vi "AuthSrpVerificationRequest_Create.vi"(7 "Header":T3, 8 "error in (no error)":errorcluster, 9 "AuthSrpVerificationRequest":T1, 10 "IRoutingSource":T2, 11 "ReplyTo":string) -> (0 "error out":errorcluster, 3 "Message":T5)   [LabVIEW 2017]
uses:
  <vilib>/addons/InsightCM/MessageBus/Base/controls/Message.ctl
  <vilib>/addons/InsightCM/MessageBus/Base/controls/MessageHeader.ctl
  <vilib>/addons/InsightCM/MessageBus/Base/controls/KeyValuePair.ctl
  <vilib>/addons/InsightCM/MessageBus/Base/controls/IRoutingSource.ctl
  <vilib>/addons/InsightCM/MessageBus/MessageLibrary/Authentication/controls/AuthSrpVerificationRequestBody.ctl
  <vilib>/addons/InsightCM/MessageBus/Base/controls/MessageClassType.ctl
  <vilib>/addons/InsightCM/Utilities/PropertyHelpers/PropertyHelpers.lvlib
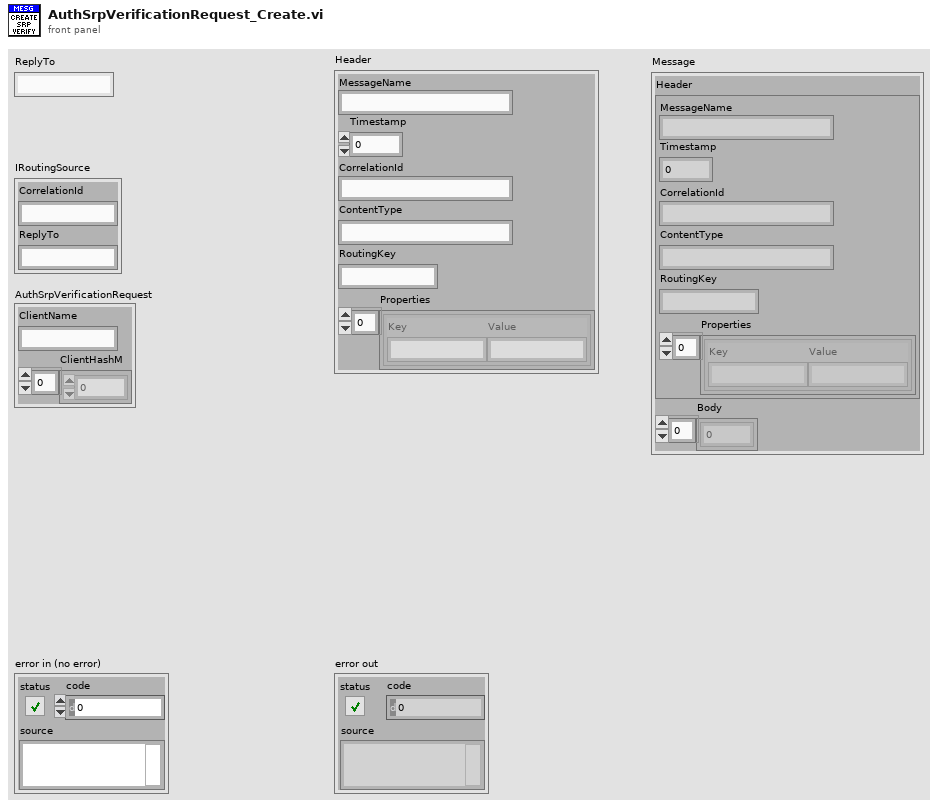
[diagram p1: front panel]
types:
  T1 = typedef "AuthSrpVerificationRequestBody.ctl" = cluster{"ClientName":string, "ClientHashM":u8[]}
  T2 = typedef "IRoutingSource.ctl" = cluster{"CorrelationId":string, "ReplyTo":string}
  T3 = typedef "MessageHeader.ctl" = cluster{"MessageName":string, "Timestamp":i64, "CorrelationId":string, "ContentType":string, "RoutingKey":string, "Properties":T4[]}
  T4 = typedef "KeyValuePair.ctl" = cluster{"Key":string, "Value":string}
  T5 = typedef "Message.ctl" = cluster{"Header":T3, "Body":u8[]}
  T6 = cluster{"ClientName":string, "ClientHashM":string}
  T7 = typedef "MessageClassType.ctl" = enum16{"Request", "Response", "Broadcast", "RoutedMessage"}
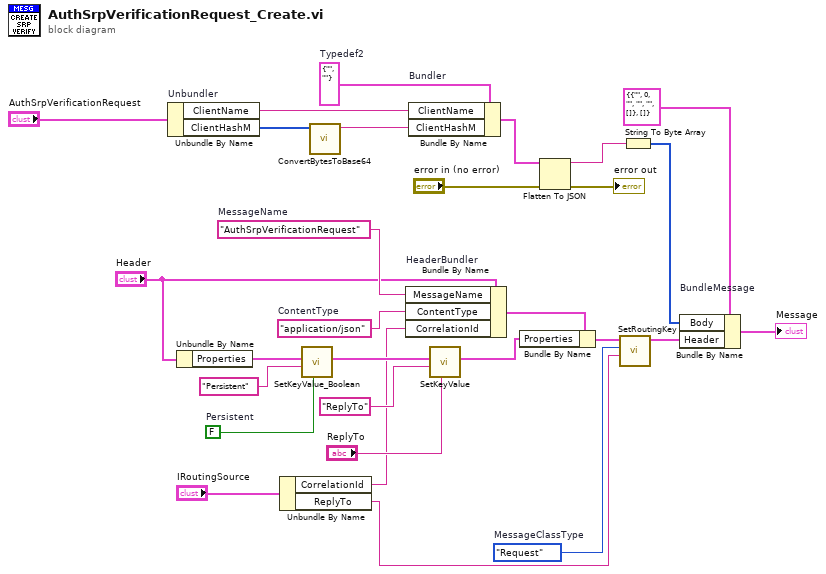
[diagram p0: block diagram]
diagram:
  w4 = T6 {"ClientName"="", "ClientHashM"=""}  # Typedef2
  w25 = MessageClassType."Request"  # MessageClassType
  w20 = FALSE  # Persistent
  w26 = "AuthSrpVerificationRequest"  # MessageName
  w23 = "application/json"  # ContentType
  n1 = Unbundle By Name "Unbundler"("AuthSrpVerificationRequest") -> ("ClientName"=w3:string, "ClientHashM"=w2:u8[])
  n2 = Unbundle By Name("Header") -> ("Properties"=w22:T4[])
  n3 = Unbundle By Name("IRoutingSource") -> ("CorrelationId"=w9:string, "ReplyTo"=w8:string)
  n4 = call <vilib>:"SetKeyValue_Boolean.vi"("value"=w20, "key"="Persistent" ("Key"), "key value pairs"=w22) -> ("key value pairs out"=w18:T4[])  [unwired: 8 in]
  n5 = call <vilib>:"ConvertBytesToBase64.vi"("U8 array"=w2) -> ("base64 encoded"=w1:string)  [unwired: 10 in]
  n6 = Bundle By Name "HeaderBundler"(cluster="Header", "MessageName"=w26, "ContentType"=w23, "CorrelationId"=w9) -> (w16:T3)
  n7 = Bundle By Name "Bundler"(cluster=w4, "ClientName"=w3, "ClientHashM"=w1) -> (w5:T6)
  n8 = call <vilib>:"SetKeyValue.vi"("value"="ReplyTo", "key"="ReplyTo" ("Key"), "key value pairs"=w18) -> ("key value pairs out"=w15:T4[])  [unwired: 8 in]
  n9 = Bundle By Name(cluster=w16, "Properties"=w15) -> (w17:T3)
  n10 = Flatten To JSON(anything=w5, error in (no error)="error in (no error)") -> (JSON string=w7:string, 11:→"error out":errorcluster)  [unwired: 1 in]
  n11 = call <vilib>:"SetRoutingKey.vi"("SendTo"=w8, "MessageClassType"=w25, "Message Header in"=w17) -> ("Message Header out"=w19:T3)  [unwired: 8 in]
  n12 = String To Byte Array(string=w7) -> (unsigned byte array=w28:u8[])
  n13 = Bundle By Name "BundleMessage"(cluster=T5 {"Header"={"MessageName"="", "Timestamp"=0, "CorrelationId"="", "ContentType"="", "RoutingKey"="", "Properties"=[]}, "Body"=[]} ("Message"), "Body"=w28, "Header"=w19) -> (→"Message":T5)
